vi "Stop Work.vi"(8 "error in (no error)":errorcluster, 11 "Spectrum Recorder in":refnum<class "Spectrum Recorder.lvclass">) -> (0 "error out":errorcluster, 3 "Spectrum Recorder out":refnum<class "Spectrum Recorder.lvclass">)   [LabVIEW 2016, in "Spectrum Recorder.lvclass"]
uses:
  Spectrum Recorder.lvclass
  C:/github/Measure_core/Worker/Worker.lvclass
  Spectrum Recorder.lvclass/Spectrum Recorder.ctl
  Measure_core/Worker/Worker.lvclass/Worker.ctl
  Measure_core/Template Module/Write Active.vi
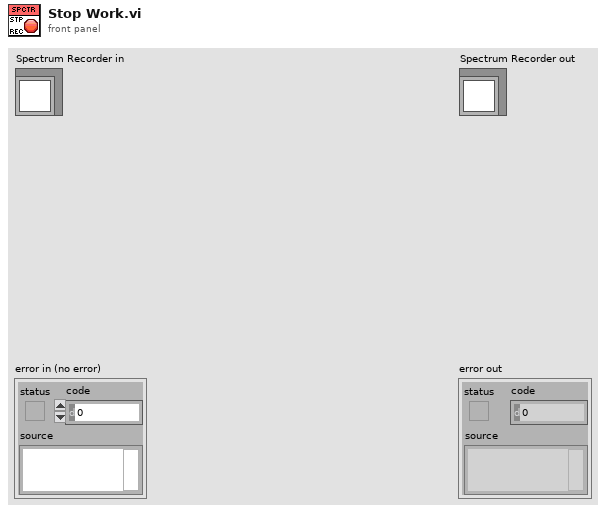
[diagram p1: front panel]
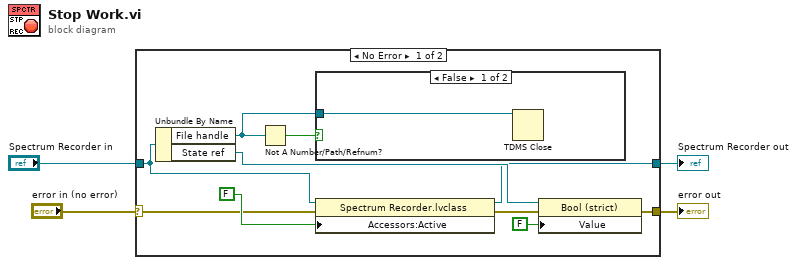
[diagram p0: block diagram]
diagram:
  n1 = case shown="No Error" "error in (no error)" {
    selector: "error in (no error)" -> [w6 w17]
    tunnel: [w11 w17] -> w3
    tunnel: [w8 w16] -> w1
    tunnel: "Spectrum Recorder in" -> [w14 w16]
    frame No Error {
      n2 = Unbundle By Name(w14) -> ("File handle"=w12:refnum<k34>, "State ref"=w9:refnum<vi>)
      n3 = Not A Number/Path/Refnum?(number/path/refnum=w12) -> (NaN/Path/Refnum?=w13:bool)
      n4 = case shown="False" w13 {
        tunnel: w12 -> [w15 _]
        frame False {
          n5 = TDMS Close(11:w15) -> ()  [unwired: 1 in, 2 out]
        }
        frame True {
        }
      }
      n6 = property class="Spectrum Recorder.lvclass"(reference=w14, error in=w6, "Accessors:Active"=FALSE ("Active")) -> (reference out=w8:refnum<class "Spectrum Recorder.lvclass">, error out=w5:errorcluster)
      n7 = property class="Bool (strict)"(reference=w9, error in=w5, "Value"=FALSE) -> (error out=w11:errorcluster)  [unwired: 1 out]
    }
    frame Error {
    }
  }
  "error out" <- w3
  "Spectrum Recorder out" <- w1
